vi "Get LPath.vi"(8 "error in (no error)":errorcluster, 10 "company name":string, 11 "license file name":string) -> (0 "error out":errorcluster, 3 "license file path":path)   [LabVIEW 2014, in "Raspberry Pi Compatible Compiler for LabVIEW.lvlib"]
doc: "Returns the path to the development license file that LabVIEW uses to activate an add-on. The location of the license file depends on the company name, because LabVIEW installs license files in the National Instruments\\Partners\\<company name>\\Licenses directory."
uses:
  <vilib>/Utility/sysdir.llb/System Directory Type.ctl
  Raspberry Pi Compatible Compiler for LabVIEW.lvlib
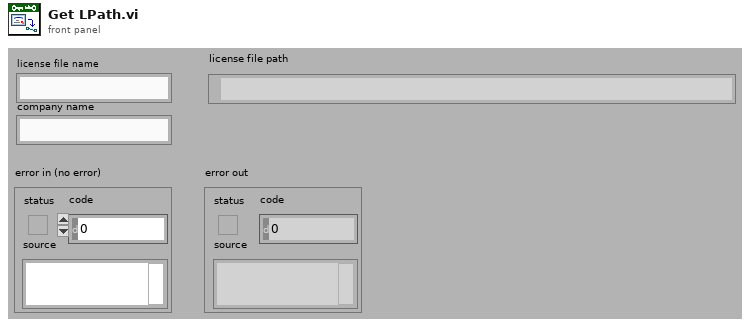
[diagram p1: front panel]
types:
  T1 = typedef "System Directory Type.ctl" = i32
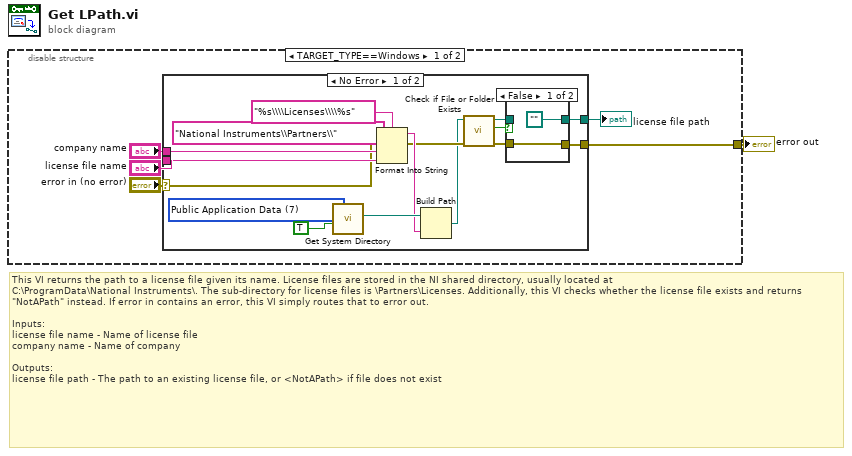
[diagram p0: block diagram]
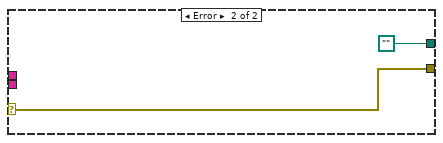
[diagram p3: hidden frame]
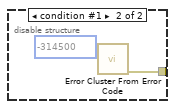
[diagram p4: hidden frame]
diagram:
  # "This VI returns the path to a license file given its name. License files are stored in the NI shared directory, usually located at\nC:\\ProgramData\\National Instruments\\. The sub-directory for license files is \\Partners\\Licenses. Additionally, this VI checks whether the license file exists and returns \"NotAPath\" instead. If error in contains an error, this VI simply routes that to error out.\n\nInputs:\nlicense file name - Name of license file\ncompany name - Name of company\n\nOutputs:\nlicense file path - The path to an existing license file, or <NotAPath> if file does not exist"
  n1 = disable-structure shown="TARGET_TYPE==Windows" {
    disable-tunnel: [w6 w30] -> w1
    frame condition #0 (active) {
      n2 = case shown="No Error" "error in (no error)" {
        selector: "error in (no error)" -> [w18 w28]
        tunnel: [w7 w28] -> w6
        tunnel: "company name" -> [w20 _]
        tunnel: "license file name" -> [w19 _]
        tunnel: [w8 path ""] -> w2
        frame No Error {
          w17 = T1 7 items=["User Home", "User Desktop", "User Documents", "User Application Data", "User Preferences", "User Temporary", "Public Documents", "Public Application Data", "Public Preferences", "System Core Libraries", "System Installed Libraries", "Application Files", "Boot Volume Root"] ("system directory type")
          n3 = call <vilib>:"Get System Directory.vi"("create directory if not found? (F)"=TRUE, "system directory type"=w17) -> ("system directory"=w15:path)  [unwired: 9 in]
          n4 = Format Into String(format string="%s\\\\Licenses\\\\%s", initial string="National Instruments\\Partners\\" ("name or relative path"), error in=w18, w20, w19) -> (resulting string=w14:string, error out=w13:errorcluster)
          n5 = Build Path(base path=w15, name or relative path=w14) -> (appended path=w12:path)
          n6 = call <vilib>:"Check if File or Folder Exists.vi"("error in (no error)"=w13, "path"=w12) -> ("error out"=w10:errorcluster, "file or folder exists?"=w11:bool, "dup path"=w9:path)  [unwired: 7 in]
          n7 = case shown="False" w11 {
            tunnel: w10 -> [w24 w25]
            tunnel: w9 -> [_ w26]
            tunnel: [path "" w26] -> w8
            tunnel: [w24 w25] -> w7
            frame False {
            }
            frame True {
            }
          }
        }
        frame Error {
        }
      }
      "license file path" <- w2
    }
    frame condition #1 {
      n8 = call <vilib>:"Error Cluster From Error Code.vi"("error code (0)"=-314500) -> ("error out"=w30:errorcluster)  [unwired: 8 in]
    }
  }
  "error out" <- w1
